vi "VI Tester Add Public Tests To TestCase.vi"(8 "error in":errorcluster, 10 "Active VI Info":T1, 11 "TestCase Refnum":refnum<vi>) -> (0 "error out":errorcluster)   [LabVIEW 2009]
uses:
  <vilib>/addons/_JKI Toolkits/RCF API/Right Click API.llb/Framework - Active VI Info - Cluster - __RightClickAPI.ctl
  <vilib>/addons/_JKI Toolkits/RCF API/Right Click API.llb/Framework - Selection Type - Enum - __RightClickAPI.ctl
  <vilib>/addons/_JKI Toolkits/RCF API/Right Click API.llb/RightClickAPI.lvlib
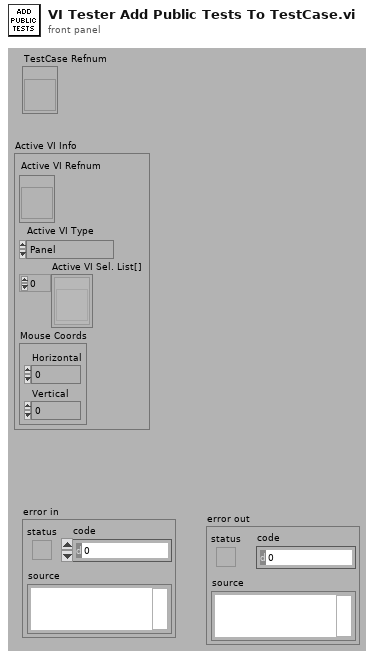
[diagram p1: front panel]
types:
  T1 = typedef "RightClickAPI.lvlib/Framework - Active VI Info - Cluster - __RightClickAPI.ctl" = cluster{"Active VI Refnum":refnum<vi>, "Active VI Type":T2, "Active VI Sel. List[]":refnum<vi>[], "Mouse Coords":cluster{"Horizontal":i32, "Vertical":i32}}
  T2 = typedef "RightClickAPI.lvlib/Framework - Selection Type - Enum - __RightClickAPI.ctl" = enum16{"Panel", "Diagram"}
  T3 = enum32{"invalid scope", "public", "private", "protected", "community"}
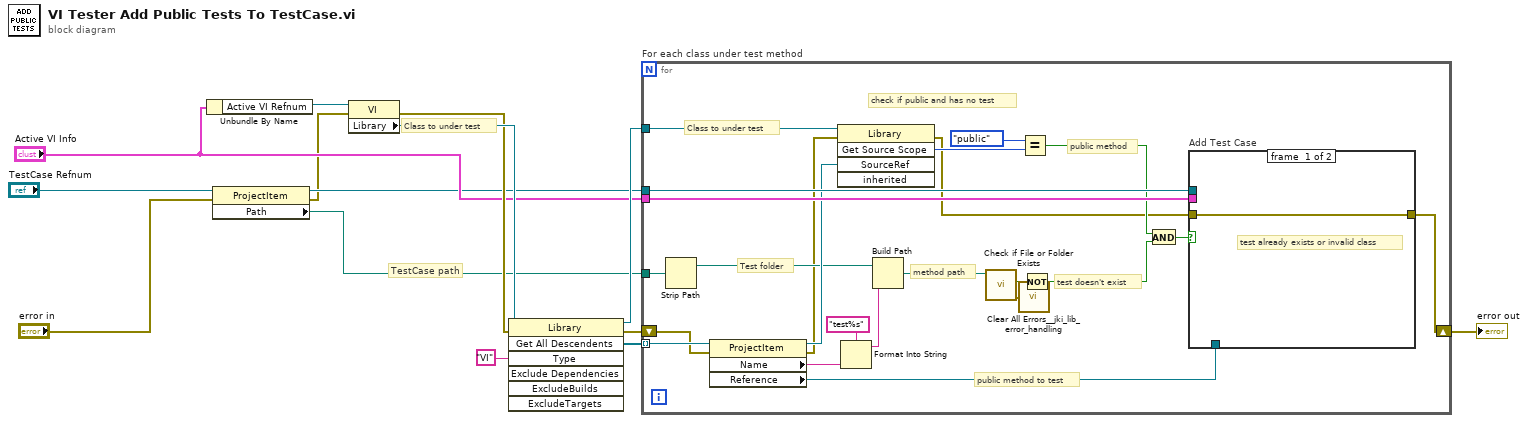
[diagram p0: block diagram]
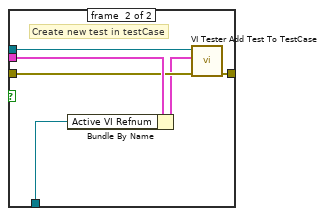
[diagram p2: hidden frame]
diagram:
  # "Class to under test"
  # "TestCase path"
  n1 = Unbundle By Name("Active VI Info") -> ("Active VI Refnum"=w10:refnum<vi>)
  n2 = property class="ProjectItem"(reference="TestCase Refnum", error in="error in") -> (reference out=w3:refnum<vi>, error out=w1:errorcluster, "Path"=w5:path)
  n3 = property class="VI"(reference=w10, error in=w1) -> (error out=w11:errorcluster, "Library"=w13:refnum<vi>)  [unwired: 1 out]
  n4 = invoke class="Library" method="Get All Descendents"(reference=w13, error in=w11, "Type"="VI") -> (reference out=w14:refnum<vi>, error out=w12:errorcluster, "All Descendents"=w8:refnum<vi>[])  [unwired: 4 in, 4 out]
  n5 = for "For each class under test method" {
    tunnel: "Active VI Info" -> [w37]
    tunnel: w3 -> [w28]
    shift-right: [w36] -> w6
    shift-left: w12 -> [w16]
    tunnel: w8 -> [w31] mode=indexing
    tunnel: w5 -> [w19]
    tunnel: w14 -> [w20]
    # "check if public and has no test"
    # "Class to under test"
    # "method path"
    # "public method to test"
    # "Test folder"
    # "public method"
    # "test doesn't exist"
    n6 = Strip Path(path=w19) -> (stripped path=w18:path)  [unwired: 1 out]
    n7 = property class="ProjectItem"(reference=w31, error in=w16) -> (reference out=w27:refnum<vi>, error out=w15:errorcluster, "Name"=w34:string, "Reference"=w29:refnum<vi>)
    n8 = invoke class="Library" method="Get Source Scope"(reference=w20, error in=w15, "SourceRef"=w27) -> (error out=w17:errorcluster, "GetSourceScope"=w26:T3)  [unwired: 2 in, 3 out]
    n9 = Format Into String(format string="test%s", w34) -> (resulting string=w33:string)  [unwired: 2 in, 1 out]
    n10 = Build Path(base path=w18, name or relative path=w33) -> (appended path=w32:path)
    n11 = call <vilib>:"Check if File or Folder Exists.vi"("path"=w32) -> ("error out"=w30:errorcluster, "file or folder exists?"=w24:bool)  [unwired: 8 in, 1 out]
    n12 = call <vilib>:"Clear All Errors__jki_lib_error_handling.vi"("error in"=w30) -> ()  [unwired: 4 in, 1 out]
    n13 = Equal?(x=T3."public", y=w26) -> (x = y?=w21:bool)
    n14 = Not(x=w24) -> (.not. x?=w23:bool)
    n15 = And(x=w21, y=w23) -> (x .and. y?=w22:bool)
    n16 = case "Add Test Case" shown="True" w22 {
      tunnel: w37 -> [_ w44]
      tunnel: w28 -> [_ w43]
      tunnel: [w38 w42] -> w36
      tunnel: w17 -> [w38 w41]
      tunnel: w29 -> [_ w39]
      frame #0 {
        # "test already exists or invalid class"
      }
      frame #1 {
        # "Create new test in testCase"
        n17 = Bundle By Name(cluster=w44, "Active VI Refnum"=w39) -> (w40:T1)
        n18 = call "VI Tester Add Test To TestCase.vi"("error in"=w41, "Active VI Info"=w40, "TestCase Refnum"=w43) -> ("error out"=w42:errorcluster)  [unwired: 8 in]
      }
    }
  }
  "error out" <- w6
